vi "Do.vi"(8 "error in (no error)":errorcluster, 10 "Actor in":refnum<class "Actor.lvclass">, 11 "Internal Message to uService Actor Core Msg":refnum<class "Internal Message to uService Actor Core Msg.lvclass">) -> (0 "error out":errorcluster, 2 "Actor out":refnum<class "Actor.lvclass">)   [LabVIEW 2026, in "TALOS.lvlib" / "Father of all uServices.lvlib" / "Internal Message to uService Actor Core Msg.lvclass"]
doc: "This VI delivers the message to the actor by calling the appropriate method(s) on the actor."
uses:
  Internal Message to uService Actor Core Msg.lvclass
  builds/Actor Framework PPL/Actor Framework.lvlibp/1abvi3w/vi.lib/ActorFramework/Actor/Actor.lvclass
  Internal Message to uService Actor Core Msg.lvclass/Internal Message to uService Actor Core Msg.ctl
  Father of all uServices/Father of all uServices.lvclass
  C:/LabVIEW Code/TALOS/builds/Actor Framework PPL/Actor Framework.lvlibp/1abvi3w/vi.lib/ActorFramework/Actor/Actor.lvclass
  Father of all uServices/Father of all uServices.lvclass/Father of all uServices.ctl
  fb889be7-b896-4491-84fe-b96acc293f92.vi
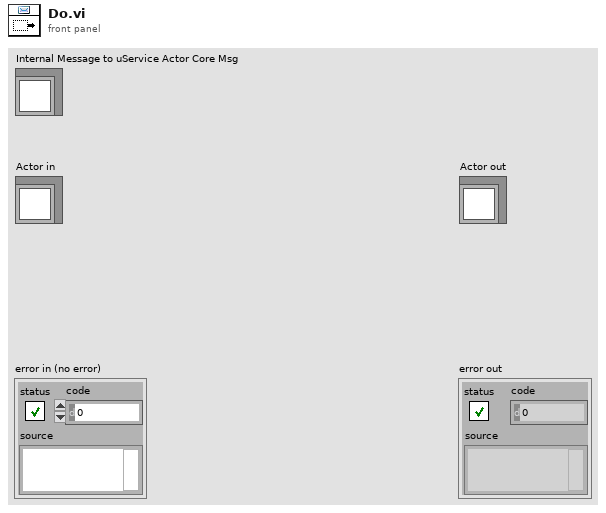
[diagram p1: front panel]
types:
  T1 = typedef "TALOS.lvlib/Father of all uServices.lvlib/Father of all uServices.lvclass/Msg to uServ Selector.ctl" = enum16{"Test string"}
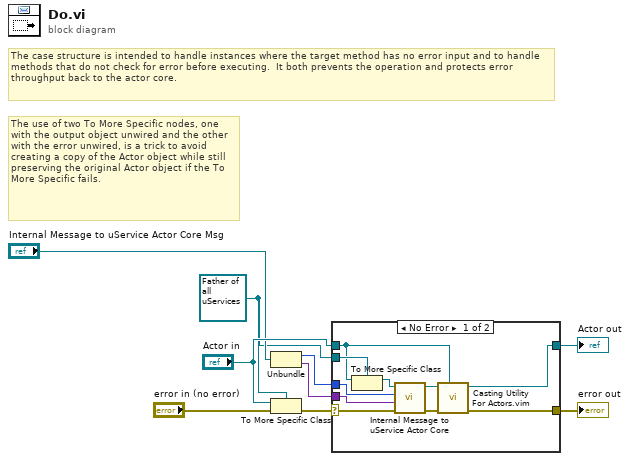
[diagram p0: block diagram]
diagram:
  w4 = refnum<class "Father of all uServices.lvclass"> refnum ("Actor in")
  # "The use of two To More Specific nodes, one with the output object unwired and the other with the error unwired, is a trick to avoid creating a copy of the Actor object while still preserving the original Actor object if the To More Specific fails."
  # "The case structure is intended to handle instances where the target method has no error input and to handle methods that do not check for error before executing.  It both prevents the operation and protects error throughput back to the actor core."
  n1 = Unbundle("Internal Message to uService Actor Core Msg") -> (w2:T1, w1:variant)
  n2 = To More Specific Class(target class=w4, reference="Actor in", error in="error in (no error)") -> (error out=w3:errorcluster)  [unwired: 1 out]
  n3 = case shown="No Error" w3 {
    selector: w3 -> [w19 w21]
    tunnel: [w13 w21] -> w9
    tunnel: [w14 w20] -> w8
    tunnel: "Actor in" -> [w16 w20]
    tunnel: w4 -> [w17 _]
    tunnel: w2 -> [w11 _]
    tunnel: w1 -> [w10 _]
    frame No Error {
      n4 = To More Specific Class(target class=w17, reference=w16) -> (specific class reference=w18:refnum<class "Father of all uServices.lvclass">)  [unwired: 1 in, 1 out]
      n5 = call "Internal Message to uService Actor Core.vi"("error in (no error)"=w19, "Message"=w10, "Msg Selector"=w11, "uService Template in"=w18) -> ("error out"=w12:errorcluster, "uService Template out"=w15:refnum<class "Father of all uServices.lvclass">)  [unwired: 6 in]
      n6 = call "Casting Utility For Actors.vim"("type"=w16, "error in (no error)"=w12, "Actor in"=w15) -> ("error out"=w13:errorcluster, "Actor out"=w14:refnum<class "Actor.lvclass">)  [unwired: 7 in]
    }
    frame Error {
      # "If type check fails, pass the original object out again."
    }
  }
  "error out" <- w9
  "Actor out" <- w8
